vi "Sea-Level SWI Write Bit.vi"(6 "Access Mode (Relative)":T1, 7 "Adapter Info":T2, 8 "error in (no error)":errorcluster, 9 "State":bool, 10 "Bit Number":u32, 11 "Handle":i32) -> (0 "error out":errorcluster, 3 "Handle Out":i32, 4 "Error Code":T3)   [LabVIEW 2011]
uses:
  TypeDefs/Sea-Level SWI Error Code.ctl
  TypeDefs/Sea-Level SWI Adapter Info.ctl
  TypeDefs/Sea-Level SWI Access Mode.ctl
  SeaIo32.dll
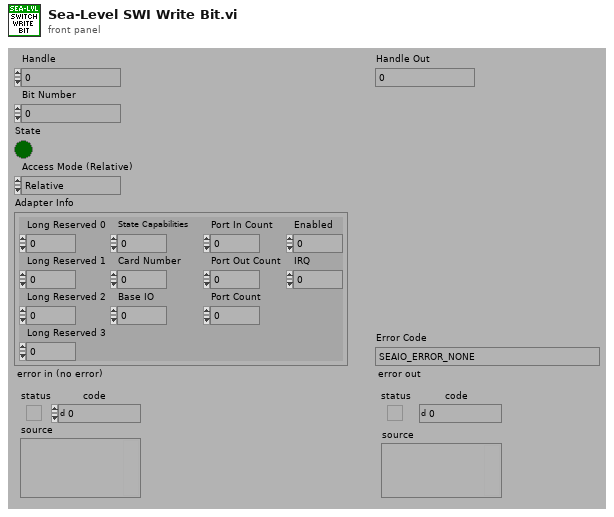
[diagram p1: front panel]
types:
  T1 = typedef "Sea-Level SWI Access Mode.ctl" = enum16{"Relative", "Absolute"}
  T2 = typedef "Sea-Level SWI Adapter Info.ctl" = cluster{"Long Reserved 0":i32, "Long Reserved 1":i32, "Long Reserved 2":i32, "Long Reserved 3":i32, "State Capabilities":i32, "Card Number":i16, "Base IO":i16, "Port In Count":i8, "Port Out Count":i8, "Port Count":i8, "Enabled":i8, "IRQ":i16}
  T3 = typedef "Sea-Level SWI Error Code.ctl" = enum16{"SEAIO_ERROR_NONE", "SEAIO_ERROR_PARAM", "SEAIO_ERROR_NOT_SUPPORTED", "SEAIO_ERROR_PORT_NOT_OPEN", "SEAIO_ERROR_INVALID_NAME", "SEAIO_ERROR_SHARING_VIOLATION", "SEAIO_ERROR_DRIVER_TYPE", "SEAIO_ERROR_BUFFER", "SEAIO_ERROR_INCOMPLETE", "SEAIO_ERROR_GENERAL", "SEAIO_ERROR_IO_PENDING", "SEAIO_ERROR_NO_TXBUFFER", "SEAIO_ERROR_INVALID_DEVICE_REQUEST", "SEAIO_ERROR_INVALID_HANDLE", "SEAIO_ERROR_CANCELED", "SEAIO_ERROR_LAST", "SEAIO_ERROR_NO_MEMORY", "SEAIO_ERROR_BUSY"}
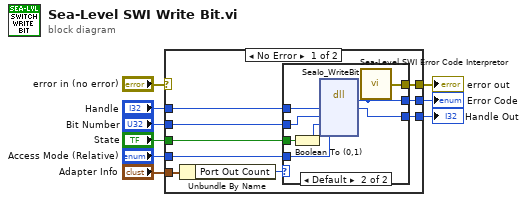
[diagram p0: block diagram]
diagram:
  n1 = case shown="No Error" "error in (no error)" {
    selector: "error in (no error)" -> [_ w27]
    tunnel: [w18 _] -> w9
    tunnel: [w17 w27] -> w8
    tunnel: "Handle" -> [w16 _]
    tunnel: "Adapter Info" -> [w15 _]
    tunnel: [w14 _] -> w4
    tunnel: "Bit Number" -> [w10 _]
    tunnel: "State" -> [w11 _]
    tunnel: "Access Mode (Relative)" -> [w12 _]
    frame No Error {
      n2 = Unbundle By Name(w15) -> ("Port Out Count"=w13:i8)
      n3 = case shown="Default" w13 {
        tunnel: [_ w26] -> w18
        tunnel: [_ w25] -> w17
        tunnel: w16 -> [_ w24]
        tunnel: [_ w23] -> w14
        tunnel: w12 -> [_ w19]
        tunnel: w11 -> [_ w21]
        tunnel: w10 -> [_ w22]
        frame 0 {
        }
        frame Default {
          n4 = Boolean To (0,1)(Boolean=w21) -> (0, 1=w20:i16)
          n5 = dll-call lib="C:/Development/Spartan/www/drivers/SWI/Sea-Level/SeaIo32.dll" fn="SeaIo_WriteBit"("Handle"=w24, "Bit Number"=w22, "State"=w20, "Access Mode"=w19) -> ("Error Code"=w26:i32, "Handle"=w23:i32)  [unwired: 5 in, 3 out]
          n6 = call "Sea-Level SWI Error Code Interpretor.vi"("Error Code"=w26) -> ("error out"=w25:errorcluster)
        }
      }
    }
    frame Error {
    }
  }
  "Error Code" <- w9
  "error out" <- w8
  "Handle Out" <- w4
